vi "Test_Exe_Main.vi"(8 "error in (no error)":errorcluster, 11 "Project Path":path=path "C:/Current projects/WS/LV32.2020..ProjectBuilder/Test/Test_Exe.lvproj") -> (0 "error out":errorcluster)   [LabVIEW 2020]
uses:
  PPL/HDH.ProjectBuilder.lvlibp
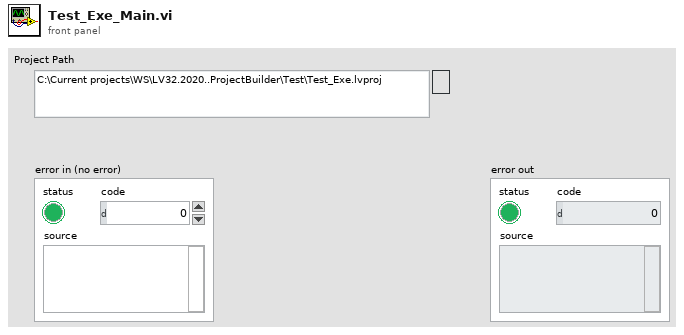
[diagram p1: front panel]
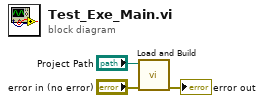
[diagram p0: block diagram]
diagram:
  n1 = call "Load and Build.vi"("error in (no error)"="error in (no error)", "Project Path"="Project Path") -> ("error out"=→"error out":errorcluster)  [unwired: 7 in, 2 out]
